vi "MACBIN Resource File Info__ogtk.vi"(6 "comment":string, 7 "write (F)":bool, 8 "error in (no error)":errorcluster, 9 "file info":T1 {"mod date" format="%<%H:%M:%S\n%m/%d/%Y>T"; "creation date" format="%<%H:%M:%S\n%m/%d/%Y>T"}, 10 "resource file":path, 11 "data file":path) -> (0 "error out":errorcluster, 1 "file info out":T1 {"mod date" format="%<%H:%M:%S\n%m/%d/%Y>T"; "creation date" format="%<%H:%M:%S\n%m/%d/%Y>T"}, 2 "resource refnum":refnum<file>, 3 "data refnum":refnum<file>, 4 "comment out":string)   [LabVIEW 2011]
uses:
  MACBIN Resource Header__ogtk.ctl
  file/file.llb/Valid Path - Traditional__ogtk.vi
panel:
  # "Please visit http://www.OpenG.org to learn about the\nOpen Source LabVIEW software movement.\n\nNOTICE -- YOU MUST LEAVE THIS NOTICE IN PLACE.  PER THE TERMS OF THE LICENSE BELOW, YOU MAY SUBLICENSE THIS SOFTWARE \nIN ANY WAY THAT DOES NOT CONFLICT WITH THIS LICENSE.\n\n### BSD License (http://www.opensource.org/licenses/bsd-license.php) Begin ###\n \nCopyright (C) 2002 Christophe Salzmann christophe.salzmann@epfl.ch\nCopyright (C) 2002-2006 Rolf Kalbermatter rolf.kalbermatter@citengineering.com\n\nAll rights reserved.\n\nRedistribution and use in source and binary forms, with or without modification, are permitted provided that the following conditions are met:\n\n    * Redistributions of source code must retain the above copyright notice, this list of conditions and the following disclaimer.\n    * Redistributions in binary form must reproduce the above copyright notice, this list of conditions and the following disclaimer in the \n       documentation and/or other materials provided with the distribution.\n    * Neither the name of SciWare, James Kring, Inc., nor the names of its contributors may be used to endorse or promote products derived \n       from this software without specific prior written permission.\n\nTHIS SOFTWARE IS PROVIDED BY THE COPYRIGHT HOLDERS AND CONTRIBUTORS \"AS IS\" AND ANY EXPRESS OR IMPLIED WARRANTIES, \nINCLUDING, BUT NOT LIMITED TO, THE IMPLIED WARRANTIES OF MERCHANTABILITY AND FITNESS FOR A PARTICULAR PURPOSE ARE \nDISCLAIMED. IN NO EVENT SHALL THE COPYRIGHT OWNER OR CONTRIBUTORS BE LIABLE FOR ANY DIRECT, INDIRECT, INCIDENTAL,\n SPECIAL, EXEMPLARY, OR CONSEQUENTIAL DAMAGES (INCLUDING, BUT NOT LIMITED TO, PROCUREMENT OF SUBSTITUTE GOODS OR \nSERVICES; LOSS OF USE, DATA, OR PROFITS; OR BUSINESS INTERRUPTION) HOWEVER CAUSED AND ON ANY THEORY OF LIABILITY, \nWHETHER IN CONTRACT, STRICT LIABILITY, OR TORT (INCLUDING NEGLIGENCE OR OTHERWISE) ARISING IN ANY WAY OUT OF THE USE \nOF THIS SOFTWARE, EVEN IF ADVISED OF THE POSSIBILITY OF SUCH DAMAGE.\n\n### BSD License End ###"
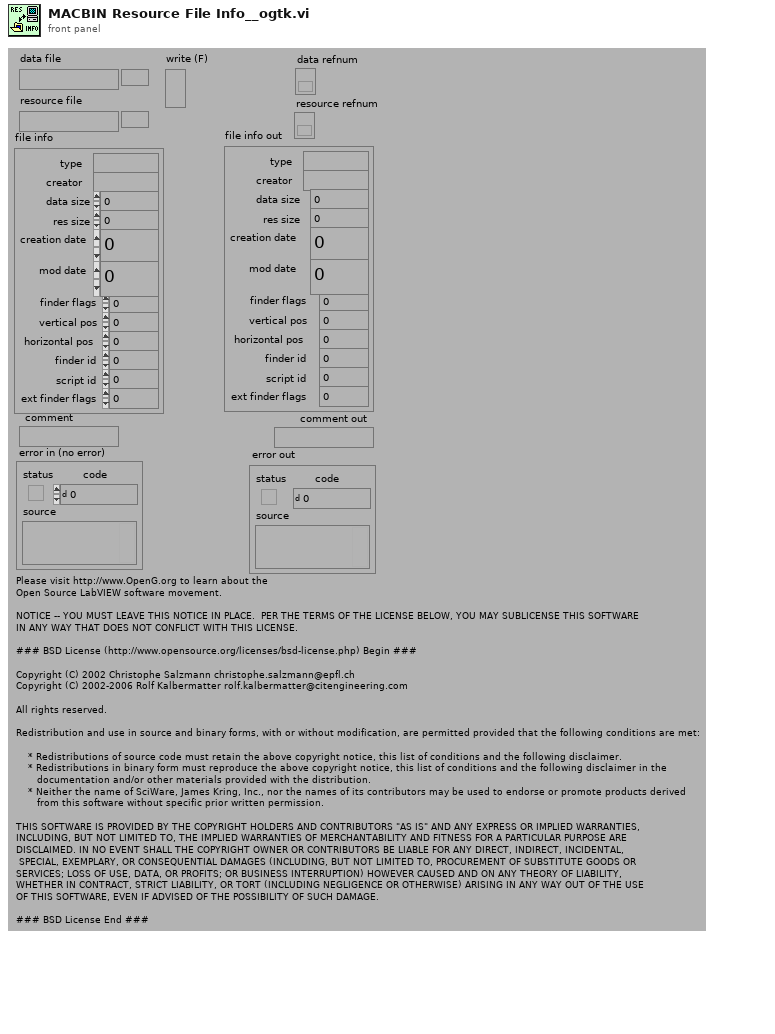
[diagram p1: front panel]
types:
  T1 = typedef "MACBIN Resource Header__ogtk.ctl" = cluster{"type":string, "creator":string, "data size":u32, "res size":u32, "creation date":u32, "mod date":u32, "finder flags":u16, "vertical pos":i16, "horizontal pos":i16, "finder id":u16, "script id":u8, "ext finder flags":u8}
  T2 = enum32{"invalid OS target", "Mac OS", "Windows 3.1", "Windows 95/NT", "Solaris 1", "Solaris 2", "HP-UX", "PowerMAX", "Linux", "Irix", "Rhapsody", "BeOS", "AIX", "OSF1", "VxWorks", "PharLap", "Carbon", "RTX", "Windows x64", "Linux x64"}
  T3 = enum16{"read/write", "read-only", "write-only", "write-only (truncate)"}
  T4 = enum16{"open", "replace", "create", "open or create", "replace or create", "replace or create with confirmation"}
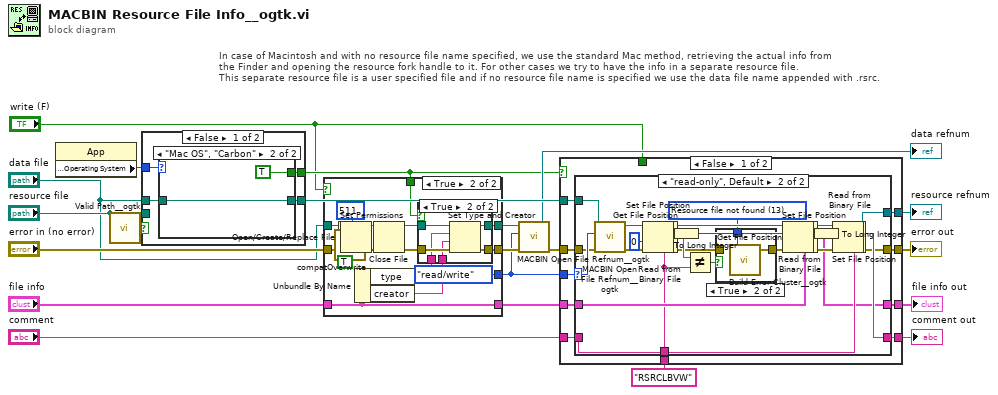
[diagram p0: block diagram]
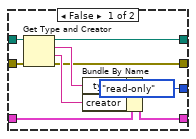
[diagram p2: hidden frame]
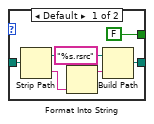
[diagram p4: hidden frame]
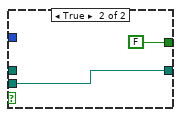
[diagram p5: hidden frame]
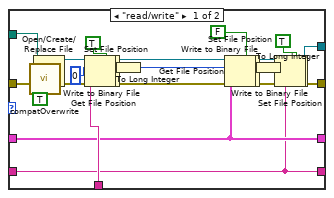
[diagram p6: hidden frame]
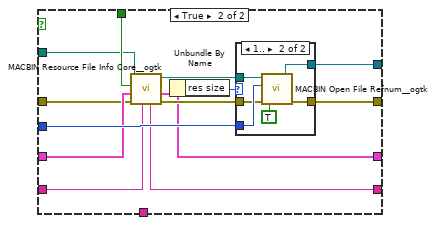
[diagram p8: hidden frame]
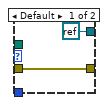
[diagram p9: hidden frame]
diagram:
  # "In case of Macintosh and with no resource file name specified, we use the standard Mac method, retrieving the actual info from\nthe Finder and opening the resource fork handle to it. For other cases we try to have the info in a separate resource file.\nThis separate resource file is a user specified file and if no resource file name is specified we use the data file name appended with .rsrc."
  n1 = property class="App"() -> ("Application:Target:Operating System"=w20:T2)  [unwired: 2 in, 2 out]
  n2 = call-poly "Valid Path__ogtk.vi"("path"="resource file") -> ("valid"=w21:bool)
  n3 = case shown="False" w21 {
    tunnel: "resource file" -> [_ w36]
    tunnel: [w25 w36] -> w18
    tunnel: "data file" -> [w24 _]
    tunnel: [w23 FALSE] -> w2
    tunnel: w20 -> [w22 _]
    frame False {
      n4 = case shown="\"Mac OS\", \"Carbon\"" w22 {
        tunnel: [w29 w34] -> w25
        tunnel: w24 -> [w27 w34]
        tunnel: [FALSE TRUE] -> w23
        frame Default {
          n5 = Strip Path(path=w27) -> (stripped path=w30:path, name=w32:string)
          n6 = Format Into String(format string="%s.rsrc" ("Format String"), w32) -> (resulting string=w31:string)  [unwired: 2 in, 1 out]
          n7 = Build Path(base path=w30, name or relative path=w31) -> (appended path=w29:path)
        }
        frame "Mac OS", "Carbon" {
        }
      }
    }
    frame True {
    }
  }
  n8 = case shown="True" "write (F)" {
    tunnel: [w37 w54] -> w8
    tunnel: "data file" -> [w43 w62]
    tunnel: "error in (no error)" -> [w44 w61]
    tunnel: [T3."read-only" ("open mode (0)") T3."read/write" ("open mode (0)")] -> w4
    tunnel: "file info" -> [w41 w52]
    tunnel: [w40 w52] -> w9
    tunnel: [w42 w53] -> w6
    tunnel: w2 -> [_ w49]
    frame False {
      n9 = Get Type and Creator(4:w44, 7:w43) -> (0:w37:errorcluster, 1:w38:string, 2:w39:string, 3:w42:path)
      n10 = Bundle By Name(cluster=w41, "type"=w39, "creator"=w38) -> (w40:T1)
    }
    frame True {
      n11 = call <vilib>:"compatOverwrite.vi"("overwrite (F)"=TRUE) -> ("overwrite?"=w46:T4)
      n12 = Open/Create/Replace File(file path (use dialog)=w62, error in=w61, operation (0:open)=w46) -> (refnum out=w57:refnum<file>, error out=w47:errorcluster)  [unwired: 3 in, 1 out]
      n13 = Set Permissions(7:i16 511 ("permissions"), 8:w47, 11:w62) -> (0:w58:errorcluster)  [unwired: 2 in, 1 out]
      n14 = Unbundle By Name(w52) -> ("type"=w51:string, "creator"=w50:string)
      n15 = Close File(refnum=w57, error in=w58) -> (path=w56:path, error out=w55:errorcluster)
      n16 = case shown="True" w49 {
        tunnel: w56 -> [w64 w70]
        tunnel: w55 -> [w63 w69]
        tunnel: [w63 w68] -> w54
        tunnel: [w64 w67] -> w53
        tunnel: w51 -> [_ w66]
        tunnel: w50 -> [_ w65]
        frame False {
        }
        frame True {
          n17 = Set Type and Creator(4:w69, 5:w65, 6:w66, 7:w70) -> (0:w68:errorcluster, 3:w67:path)
        }
      }
    }
  }
  n18 = call "MACBIN Open File Refnum__ogtk.vi"("error in (no error)"=w8, "open mode (0)"=w4, "file path"=w6) -> ("error out"=w7:errorcluster, "file refnum"=→"data refnum":refnum<file>)  [unwired: 4 in]
  n19 = case shown="False" w2 {
    tunnel: [w79 w164] -> w17
    tunnel: [w80 w163] -> w13
    tunnel: w18 -> [w77 w154]
    tunnel: w4 -> [w78 w162]
    tunnel: w7 -> [w76 w155]
    tunnel: w9 -> [w75 w161]
    tunnel: [w74 w153] -> w15
    tunnel: "comment" -> [w73 w160]
    tunnel: [w72 w159] -> w14
    tunnel: "RSRCLBVW" -> [w71 _]
    tunnel: "write (F)" -> [_ w158]
    frame False {
      n20 = case shown="\"read-only\", Default" w78 {
        selector: w78 -> [_ w129]
        tunnel: [w106 w131] -> w80
        tunnel: [w105 w132] -> w79
        tunnel: w77 -> [w113 w148]
        tunnel: w76 -> [w97 w128]
        tunnel: w75 -> [w96 w144]
        tunnel: [w96 w130] -> w74
        tunnel: w73 -> [w95 w143]
        tunnel: [w95 w142] -> w72
        tunnel: w71 -> [w99 w137]
        frame "read/write" {
          n21 = call <vilib>:"compatOverwrite.vi"("overwrite (F)"=TRUE) -> ("overwrite?"=w81:T4)
          n22 = Open/Create/Replace File(file path (use dialog)=w113, error in=w97, operation (0:open)=w81) -> (refnum out=w107:refnum<file>, error out=w111:errorcluster)  [unwired: 3 in, 1 out]
          n23 = Set File Position(offset (in bytes) (0)=0 ("pos offset (0)"), refnum=w107, error in=w111) -> (refnum out=w86:refnum<file>, error out=w85:errorcluster)  [unwired: 1 in]
          n24 = Write to Binary File(file (use dialog)=w86, data=w99, error in=w85, 5:TRUE ("header (F)")) -> (refnum out=w84:refnum<file>, error out=w83:errorcluster)  [unwired: 2 in, 1 out]
          n25 = Get File Position(4:w83, 7:w84) -> (0:w100:errorcluster, 2:w82:i64, 3:w108:refnum<file>)
          n26 = To Long Integer(number=w82) -> (32bit integer=w102:i32)
          n27 = Set File Position(offset (in bytes) (0)=w102, refnum=w108, error in=w100) -> (refnum out=w94:refnum<file>, error out=w93:errorcluster)  [unwired: 1 in]
          n28 = Write to Binary File(file (use dialog)=w94, data=w96, error in=w93, 5:FALSE ("prepend array or string size? (T)")) -> (refnum out=w92:refnum<file>, error out=w91:errorcluster)  [unwired: 2 in, 1 out]
          n29 = Get File Position(4:w91, 7:w92) -> (0:w110:errorcluster, 2:w90:i64, 3:w109:refnum<file>)
          n30 = To Long Integer(number=w90) -> (32bit integer=w104:i32)
          n31 = Set File Position(offset (in bytes) (0)=w104, refnum=w109, error in=w110) -> (refnum out=w88:refnum<file>, error out=w87:errorcluster)  [unwired: 1 in]
          n32 = Write to Binary File(file (use dialog)=w88, data=w95, error in=w87, 5:TRUE ("header (F)")) -> (refnum out=w105:refnum<file>, error out=w106:errorcluster)  [unwired: 2 in, 1 out]
        }
        frame "read-only", Default {
          w133 = 13 items=["No error", "Argument error", "Memory is full", "Out of zone", "End of file", "File already open", "Generic file I/O error", "File not found", "File permission error", "Disk is full", "Duplicate path", "Too many files open", "System feature not enabled", "Resource file not found", "Cannot add resource", "Resource not found", "Image not found", "Image memory error", "Pen does not exist", "Config type invalid", "Config token not found", "Config parse error", "Config memory error", "Bad external code format", "Bad external code offset", "External code not present", "Null window", "Destroy window error", "Null menu", "Print aborted", "Bad print record", "Print driver error", "Windows error during printing", "Memory error during printing", "Print dialog error", "Generic print error", "Invalid device refnum", "Device not found", "Device parameter error", "Device unit error", "Cannot open device", "Device call aborted", "Generic error", "Cancelled by user", "Object ID too low", "Object ID too high", "Object not in heap", "Unknown heap", "Unknown object (invalid DefProc)", "Unknown object (DefProc not in table)", "Message out of range", "Invalid (null) method", "Unknown message", "Manager call not supported", "Bad address", "Network operation in progress", "Network operation timed out", "Connection is busy", "Network attribute not supported", "Network error", "Address in use", "System out of memory", "Connection aborted", "Connection refused", "Not connected", "Already connected", "Connection closed", "Initialization error (interapplication manager)", "Bad occurrence", "Wait on unbound occurrence handler", "Occurrence queue overflow", "Datalog type conflict", "Unused", "Unrecognized type (interapplication manager)", "Memory corrupt", "Failed to make temporary DLL", "Old CIN version", "Drag socket not found", "Failed to load drop-object", "Failed to register OLE object", "Failed to release OLE object", "Format specifier type mismatch", "Unknown format specifier", "Too few format specifiers", "Too many format specifiers", "Scan failed", "Newer CIN version", "Error converting to variant", "Runtime menu error", "Password tampered", "Variant attribute not found", "Incompatible variant data type", "Event data is not available", "Event Store is not present", "Occurrence is not found", "Event Queue is not created", "Event info is not available", "Refnum passed is NULL", "Error retrieving Class GUID", "Error retrieving CoClass GUID", "Error retrieving TypeLib GUID.", "Bad built application magic bytes.", "Specific driver is different from the specific driver associated with the Logical Name.", "There is no session opened to the class driver.", "Max Error", "MAX - Error with config objects", "MAX - Error loading configuration", "MAX - Group not supported"]
          n33 = call "MACBIN Open File Refnum__ogtk.vi"("error in (no error)"=w128, "open mode (0)"=w129, "file path"=w148) -> ("error out"=w127:errorcluster, "file refnum"=w126:refnum<file>)  [unwired: 4 in]
          n34 = Set File Position(offset (in bytes) (0)=0 ("pos offset (0)"), refnum=w126, error in=w127) -> (refnum out=w118:refnum<file>, error out=w117:errorcluster)  [unwired: 1 in]
          n35 = Read from Binary File(5:w137, 8:w117, 11:w118) -> (0:w115:errorcluster, 2:w138:string, 3:w116:refnum<file>)  [unwired: 3 in, 1 out]
          n36 = Get File Position(4:w115, 7:w116) -> (0:w135:errorcluster, 2:w114:i64, 3:w147:refnum<file>)
          n37 = To Long Integer(number=w114) -> (32bit integer=w140:i32)
          n38 = Not Equal?(x=w138, y=w137) -> (x != y?=w136:bool)
          n39 = case shown="True" w136 {
            tunnel: w135 -> [w149 _]
            tunnel: [w149 w151] -> w134
            tunnel: w133 -> [_ w150]
            frame False {
            }
            frame True {
              n40 = call "Build Error Cluster__ogtk.vi"("code"=w150) -> ("error out"=w151:errorcluster)  [unwired: 1 in]
            }
          }
          n41 = Set File Position(offset (in bytes) (0)=w140, refnum=w147, error in=w134) -> (refnum out=w123:refnum<file>, error out=w122:errorcluster)  [unwired: 1 in]
          n42 = Read from Binary File(5:w144, 8:w122, 11:w123) -> (0:w120:errorcluster, 2:w130:T1, 3:w121:refnum<file>)  [unwired: 3 in, 1 out]
          n43 = Get File Position(4:w120, 7:w121) -> (0:w145:errorcluster, 2:w119:i64, 3:w146:refnum<file>)
          n44 = To Long Integer(number=w119) -> (32bit integer=w141:i32)
          n45 = Set File Position(offset (in bytes) (0)=w141, refnum=w146, error in=w145) -> (refnum out=w125:refnum<file>, error out=w124:errorcluster)  [unwired: 1 in]
          n46 = Read from Binary File(5:w143, 8:w124, 11:w125) -> (0:w131:errorcluster, 2:w142:string, 3:w132:refnum<file>)  [unwired: 3 in, 1 out]
        }
      }
    }
    frame True {
      n47 = call "MACBIN Resource File Info Core__ogtk.vi"("comment"=w160, "error in (no error)"=w155, "file info in"=w161, "write (F)"=w158, "resource file"=w154) -> ("error out"=w157:errorcluster, "file info out"=w153:T1, "resource file out"=w156:path, "comment out"=w159:string)  [unwired: 1 out]
      n48 = Unbundle By Name(w153) -> ("res size"=w152:u32)
      n49 = case shown="1.." w152 {
        tunnel: [refnum<k0> refnum w172] -> w164
        tunnel: [w166 w171] -> w163
        tunnel: w162 -> [_ w170]
        tunnel: w157 -> [w166 w169]
        tunnel: w156 -> [_ w168]
        frame Default {
        }
        frame 1.. {
          n50 = call "MACBIN Open File Refnum__ogtk.vi"("resource fork (F)"=TRUE, "error in (no error)"=w169, "open mode (0)"=w170, "file path"=w168) -> ("error out"=w171:errorcluster, "file refnum"=w172:refnum<file>)  [unwired: 3 in]
        }
      }
    }
  }
  "file info out" <- w15
  "error out" <- w13
  "comment out" <- w14
  "resource refnum" <- w17
